vi "parse headers.vi"(11 "String":string) -> (3 "headers":map{string, string[]}(c390))   [LabVIEW 2019, in "WebSocket Server Toolkit.lvlib"]
uses:
  WebSocket Server Toolkit.lvlib
  <vilib>/Utility/miscctls.llb/LVMapReplaceAction.ctl
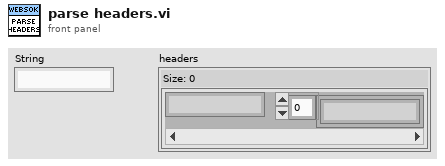
[diagram p1: front panel]
types:
  T1 = typedef "LVMapReplaceAction.ctl" = enum32{"Modify Entry only if found", "Add or Modify Entry", "Delete Entry"}
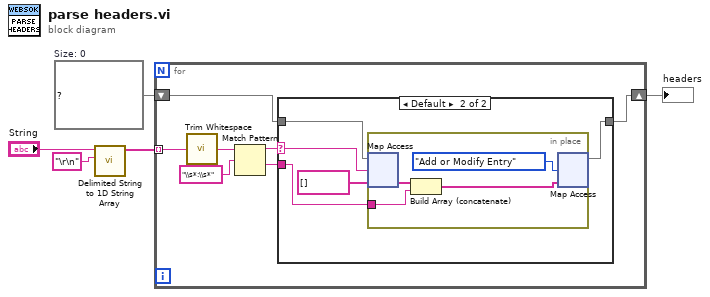
[diagram p0: block diagram]
diagram:
  w5 = map{string, string[]} {}  # Size: 0
  n1 = call <vilib>:"Delimited String to 1D String Array.vi"("delimiter"="\r\n" ("delimited string"), "delimited string"="String") -> ("string array"=w4:string[])  [unwired: 9 in]
  n2 = for {
    tunnel: w4 -> [w12] mode=indexing
    shift-right: [w7] -> w1
    shift-left: w5 -> [w8]
    n3 = call <vilib>:"Trim Whitespace.vi"("string"=w12) -> ("trimmed string"=w11:string)  [unwired: 1 in]
    n4 = Match Pattern(string=w11, regular expression="\\s*:\\s*") -> (before substring=w6:string, after substring=w9:string)  [unwired: 1 in, 2 out]
    n5 = case shown="Default" w6 {
      selector: w6 -> [_ w17]
      tunnel: w9 -> [_ w15]
      tunnel: w8 -> [w13 w18]
      tunnel: [w13 w14] -> w7
      frame "" {
      }
      frame Default {
        n6 = in-place {
          in-place-border: w15 -> [w21]
          n7 = in-place-map #1(w18, w17, string[] []) -> (w22:string[])  [unwired: 1 out]
          n8 = Build Array (concatenate)(w22, w21) -> (w20:string[])
          n9 = in-place-map #1(w20, LVMapReplaceAction."Add or Modify Entry" ("action")) -> (w14:map{string, string[]})  [unwired: 2 out]
        }
      }
    }
  }
  "headers" <- w1
